vi "user32_DragDetect.vi"(0 "hWnd":u32, 5 "Position":cluster{"x":i32, "y":i32}, 11 "错误输入（无错误）":errorcluster) -> (4 "dup hWnd":u32, 6 "OutOfRect?":bool, 15 "错误输出":errorcluster)   [LabVIEW 2011]
doc: "该函数捕获并跟踪鼠标的移动直到用户松开左键、按下Esc。键或者将鼠标移动到围绕指定点的“拖动矩形”之外。拖动矩形的宽和高由函数GetSystemMetrics返回的SM_CXDRAG或SM_CYDRAG确定。"
uses:
  user32.dll
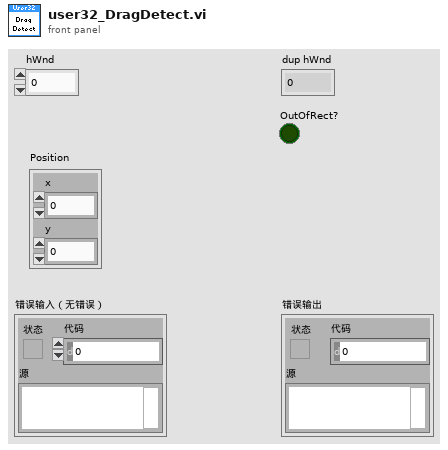
[diagram p1: front panel]
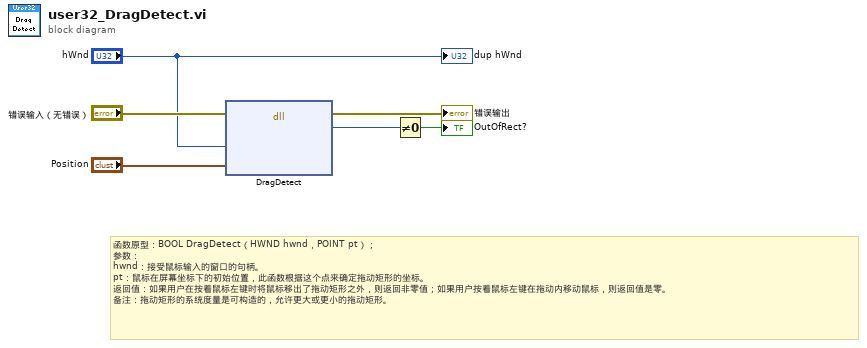
[diagram p0: block diagram]
diagram:
  # "函数原型：BOOL DragDetect（HWND hwnd，POINT pt）；\n参数：\nhwnd：接受鼠标输入的窗口的句柄。\npt：鼠标在屏幕坐标下的初始位置，此函数根据这个点来确定拖动矩形的坐标。\n返回值：如果用户在按着鼠标左键时将鼠标移出了拖动矩形之外，则返回非零值；如果用户按着鼠标左键在拖动内移动鼠标，则返回值是零。\n备注：拖动矩形的系统度量是可构造的，允许更大或更小的拖动矩形。"
  n1 = dll-call lib="user32.dll" fn="DragDetect"(error in="错误输入（无错误）", "hWnd"="hWnd", "Position"="Position") -> (error out=→"错误输出":errorcluster, "Bool"=w3:u8)  [unwired: 4 in, 1 out]
  n2 = Not Equal To 0?(x=w3) -> (x != 0?=→"OutOfRect?":bool)
  "dup hWnd" <- "hWnd"
